vi "Create OPC UA Client.vi"(8 "error in (no error)":errorcluster, 9 "update rate (1000 ms)":dbl=1000.0, 10 "port (4840)":i32=4840, 11 "URLs":string[](array[string])) -> (0 "error out":errorcluster, 2 "OPC UA data change event":refnum<user-event>, 3 "OPC UA Client.lvclass":refnum<class "OPC UA Client.lvclass">)   [LabVIEW 2016, in "OPC UA Client.lvclass"]
uses:
  OPC UA Client Class/OPC UA Client.lvclass
  OPC UA Client Class/OPC UA Client.lvclass/OPC UA Client.ctl
  <vilib>/OPCUA/NI OPC UA Client.lvlib
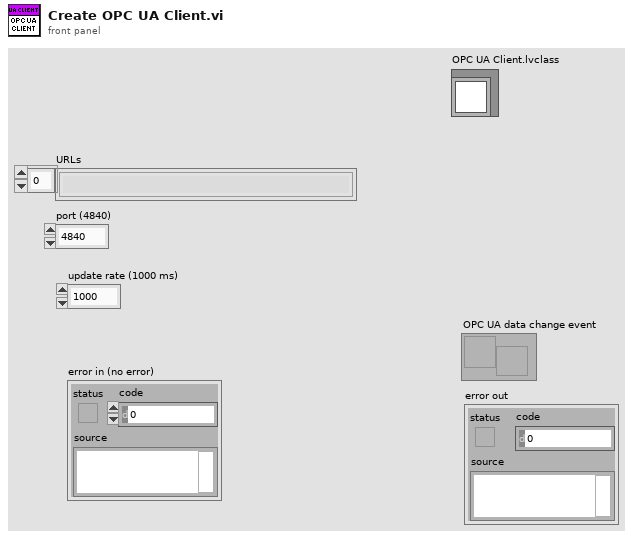
[diagram p1: front panel]
types:
  T1 = cluster{"message mode":enum16{"None", "Sign", "Sign and Encrypt"}, "security":enum16{"Basic256", "Basic128Rsa15"}}
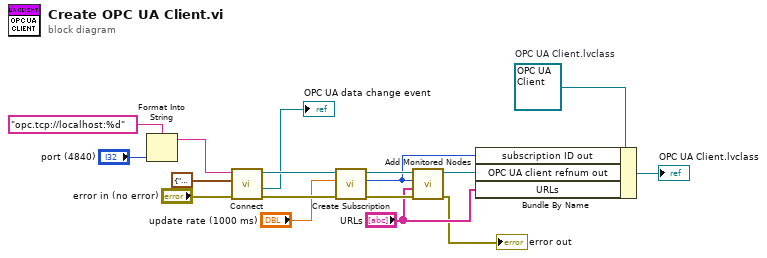
[diagram p0: block diagram]
diagram:
  w6 = refnum<class "OPC UA Client.lvclass"> refnum  # OPC UA Client.lvclass
  n1 = Format Into String(format string="opc.tcp://localhost:%d" ("server endpoint URL"), "port (4840)") -> (resulting string=w14:string)  [unwired: 2 in, 1 out]
  n2 = call <vilib>:"Connect.vi"("error in (no error)"="error in (no error)", "security policy"=T1 {"message mode"=enum."None", "security"=enum."Basic256"}, "server endpoint URL"=w14) -> ("error out"=w13:errorcluster, "OPC UA data change event"=→"OPC UA data change event":refnum<user-event>, "OPC UA client refnum out"=w11:refnum<k21>)  [unwired: 6 in]
  n3 = call <vilib>:"Create Subscription.vi"("error in (no error)"=w13, "update rate (1000 ms)"="update rate (1000 ms)", "OPC UA client refnum in"=w11) -> ("error out"=w16:errorcluster, "subscription ID out"=w5:u32, "OPC UA client refnum out"=w17:refnum<k21>)  [unwired: 6 in]
  n4 = call <vilib>:"Add Monitored Nodes.vi"("error in (no error)"=w16, "array of node path"="URLs", "subscription ID in"=w5, "OPC UA client refnum in"=w17) -> ("error out"=→"error out":errorcluster, "OPC UA client refnum out"=w4:refnum<k21>)  [unwired: 5 in, 1 out]
  n5 = Bundle By Name(cluster=w6, "subscription ID out"=w5, "OPC UA client refnum out"=w4, "URLs"="URLs") -> (→"OPC UA Client.lvclass":refnum<class "OPC UA Client.lvclass">)
